vi "SendMultipleQueueMessages.vi"(6 "timeout in ms (-1)":i32=-1, 8 "error in":errorcluster, 9 "message data []":variant[](array[variant]), 10 "message names []":string[](array[string]), 11 "message ref in":refnum<class "CLM_LocalMessage_Queue.lvclass">) -> (0 "error out":errorcluster, 3 "message ref out":refnum<class "CLM_LocalMessage_Queue.lvclass">, 4 "timed out?":bool)   [LabVIEW 2013, in "CLM_LocalMessage_Queue.lvclass"]
uses:
  CLM_LocalMessage_Queue.lvclass
  CLM_LocalMessage_Queue.lvclass/CLM_LocalMessage_Queue.ctl
  SendQueueMessage_Cluster.vi
  LocalMessage/BundleMessageCluster.vi
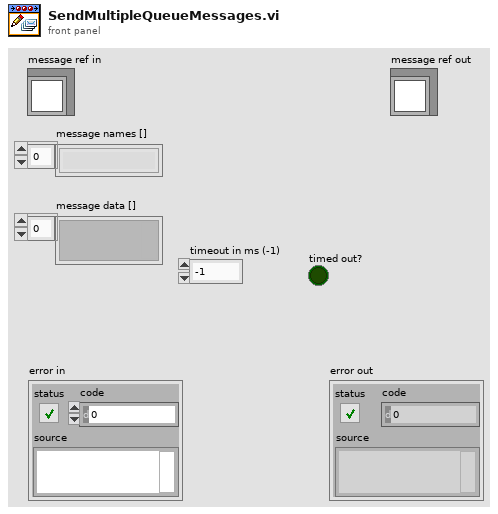
[diagram p1: front panel]
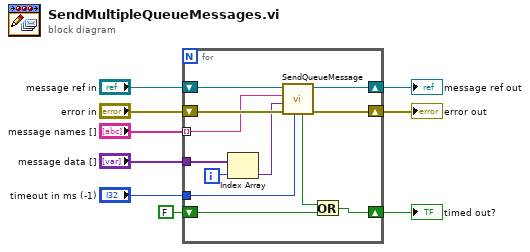
[diagram p0: block diagram]
diagram:
  n1 = for {
    shift-right: [w18] -> w3
    shift-left: "error in" -> [w21]
    shift-right: [w19] -> w4
    shift-left: "message ref in" -> [w20]
    tunnel: "message names []" -> [w17] mode=indexing
    tunnel: "message data []" -> [w16]
    tunnel: "timeout in ms (-1)" -> [w13]
    shift-right: [w11] -> w1
    shift-left: FALSE -> [w10]
    i -> [w15]
    n2 = Index Array(array=w16, index=w15) -> (element=w14:variant)
    n3 = call "SendQueueMessage.vi"("timeout in ms (-1)"=w13, "error in"=w21, "data"=w14, "name"=w17, "message ref in"=w20) -> ("error out"=w18:errorcluster, "message ref out"=w19:refnum<class "CLM_LocalMessage_Queue.lvclass">, "timed out?"=w12:bool)  [unwired: 4 in]
    n4 = Or(x=w12, y=w10) -> (x .or. y?=w11:bool)
  }
  "error out" <- w3
  "message ref out" <- w4
  "timed out?" <- w1
